vi "NMRvmeCard4.vi"() -> ()   [LabVIEW 2013]
uses:
  <vilib>/Utility/file.llb/Read From Spreadsheet File (DBL).vi
  <vilib>/Analysis/NI_AALBase.lvlib
panel:
  out "Peak center (MHz)":sgl=213.00728 format="%.3f"
  out "Peak width (MHz)":sgl=0.03243152 format="%.5f"
  in  "Max":bool=TRUE
  in  "Logoffset (V)":dbl=-5.924000000000002 min=-9.0 max=0.0 step=0.0005 format="%_5g"
  in  "Phase (V)":dbl=6.5 min=0.0 max=9.0 step=0.0005 format="%_5g"
  out "Telnet error out":errorcluster
  in  "Real/Quad Q curve":bool
  out "Temperature (C)":dbl(graph)=25.12
  out "+3V supply":dbl=3.245 format="%_4g"
  out "Temp (C)":dbl=25.12 format="%_4g"
  in  "RemovePed":bool=TRUE
  in  "IF / LOG Det":bool
  in  "Q curve file":string="realback212a.txt"
  out "File name 2":string="C:\\users\\plm\\Desktop\\rssmt\\realback212a.txt"
  in  "AutoTune":bool
  out "RF OK":bool=TRUE
  out "Peak area (V-MHz)":sgl=0.030005611 format="%.5f"
  in  "Gauss Fit":bool
  out "NMR Graph + Fit":cluster{cluster{dbl, "Numeric":dbl}[]}[](graph)=[{[{212.6, "Numeric"=-0.02921344062499997}, {212.60999999999999, "Numeric"=-0.03215714062499996}, {212.62, "Numeric"=-0.04651344062500006}, {212.63, "Numeric"=-0.03536254062499999}, {212.64, "Numeric"=-0.04138284062500002}, {212.65, "Numeric"=-0.041101840625000045}, {212.66, "Numeric"=-0.040491840625000046}, {212.67, "Numeric"=-0.026806840624999988}, {212.68, "Numeric"=-0.027852040624999956}, {212.69, "Numeric"=-0.040467640625000016}, {212.7, "Numeric"=-0.03304384062499998}, {212.71, "Numeric"=-0.031359340625}, {212.72, "Numeric"=-0.022591940624999994}, {212.73, "Numeric"=-0.01193064062500001}, {212.74, "Numeric"=-0.01354794062499997}, {212.75, "Numeric"=-0.013213040624999998}, {212.76, "Numeric"=-0.015344740624999985}, {212.77, "Numeric"=-0.00963054062500001}, {212.78, "Numeric"=-0.01998944062499996}, {212.79, "Numeric"=-0.029504540624999985}, {212.8, "Numeric"=-0.024544640624999982}, {212.81, "Numeric"=-0.024524280624999985}, {212.82, "Numeric"=-0.03563309062499998}, {212.82999999999998, "Numeric"=-0.027916150624999976}, {212.84, "Numeric"=-0.024776840624999984}, {212.85, "Numeric"=-0.018898880624999982}, {212.85999999999999, "Numeric"=-0.029138710624999974}, {212.87, "Numeric"=-0.028821390624999978}, {212.88, "Numeric"=-0.020467430624999977}, {212.89, "Numeric"=-0.017315150624999977}, {212.9, "Numeric"=-0.01772434062499998}, {212.91, "Numeric"=-0.01372252062499998}, {212.92, "Numeric"=-0.004970290624999978}, {212.93, "Numeric"=0.006207539375000022}, {212.94, "Numeric"=0.027450659375000026}, {212.95, "Numeric"=0.06105685437500003}, {212.96, "Numeric"=0.124804897375}, {212.97, "Numeric"=0.208860369375}, {212.98, "Numeric"=0.347462365375}, {212.99, "Numeric"=0.35238067957499997}, {213.0, "Numeric"=0.27427406967500007}, {213.01, "Numeric"=0.235365305375}, {213.02, "Numeric"=0.19710875937500003}, {213.03, "Numeric"=0.155801636375}, {213.04, "Numeric"=0.14391716037500002}, {213.05, "Numeric"=0.15687335037500003}, {213.06, "Numeric"=0.14626102237500002}, {213.07, "Numeric"=0.16260765937500002}, {213.08, "Numeric"=0.140506499375}, {213.09, "Numeric"=0.098470809375}, {213.1, "Numeric"=0.06081699937500002}, {213.11, "Numeric"=0.04152627937500002}, {213.12, "Numeric"=0.044080989375000025}, {213.13, "Numeric"=0.02363172937500002}, {213.14000000000001, "Numeric"=0.030902539375000024}, {213.15, "Numeric"=0.04097138937500002}, {213.16, "Numeric"=0.04776892937500001}, {213.17000000000002, "Numeric"=0.059566619375000025}, {213.18, "Numeric"=0.058962209375}, {213.19, "Numeric"=0.03914579937500002}, {213.2, "Numeric"=0.03482955937500002}, {213.21, "Numeric"=0.037365659375000006}, {213.22, "Numeric"=0.016002559375000038}, {213.23, "Numeric"=0.013610259374999996}, {213.24, "Numeric"=0.023504359375000013}, {213.25, "Numeric"=0.020751659374999988}, {213.26, "Numeric"=0.014210559374999994}, {213.27, "Numeric"=0.01739725937500001}, {213.28, "Numeric"=0.023614959374999973}, {213.29, "Numeric"=0.018911459375000002}, {213.3, "Numeric"=0.023336959374999973}, {213.31, "Numeric"=0.02134245937500002}, {213.32, "Numeric"=0.017474059375000024}, {213.33, "Numeric"=0.018297259374999993}, {213.34, "Numeric"=0.013561559374999983}, {213.35, "Numeric"=0.02328705937499998}, {213.36, "Numeric"=0.021839359374999985}, {213.37, "Numeric"=0.031837559375}, {213.38, "Numeric"=0.038417959374999984}, {213.39000000000001, "Numeric"=0.04150235937499997}, {213.4, "Numeric"=0.04535425937499999}]}]
  in  "Amp of Q curve":dbl=1.1 min=0.0 max=9.0 step=0.01 format="%_3f"
  in  "Subtract Q curve":bool=TRUE
  out "Pedestal Offset":dbl(graph)=0.028833440624999977
  out "Pedestal Difference":dbl(graph)=0.056176981249999994
  out "# Good Spectra":i32=994
  in  "Quality cuts":bool=TRUE
  out "Pedestal OK":bool=TRUE
  out "Sweep #":i32=6
  out "1st Sweep":bool
  out "ADC volts OK":bool=TRUE
  out "Peak Height Distribution":cluster{"Y":dbl[], "Y":dbl[]}[](graph)=[{"Y"=[0.6224574999999992, 0.6237974999999992, 0.6251374999999992, 0.6264774999999992, 0.6278174999999993, 0.6291574999999993, 0.6304974999999993, 0.6318374999999993, 0.6331774999999993, 0.6345174999999993, 0.6358574999999993, 0.6371974999999993, 0.6385374999999993, 0.6398774999999993, 0.6412174999999992, 0.6425574999999992, 0.6438974999999992, 0.6452374999999992, 0.6465774999999993, 0.6479174999999993, 0.6492574999999993, 0.6505974999999993, 0.6519374999999993, 0.6532774999999993, 0.6546174999999993, 0.6559574999999993, 0.6572974999999993, 0.6586374999999993, 0.6599774999999993, 0.6613174999999992, 0.6626574999999992, 0.6639974999999992, 0.6653374999999992, 0.6666774999999993, 0.6680174999999993, 0.6693574999999993, 0.6706974999999993, 0.6720374999999993, 0.6733774999999993, 0.6747174999999993, 0.6760574999999993, 0.6773974999999993, 0.6787374999999993, 0.6800774999999992, 0.6814174999999992, 0.6827574999999992, 0.6840974999999992, 0.6854374999999993, 0.6867774999999993, 0.6881174999999993, 0.6894574999999993, 0.6907974999999993, 0.6921374999999993, 0.6934774999999993, 0.6948174999999993, 0.6961574999999993, 0.6974974999999993, 0.6988374999999992, 0.7001774999999992, 0.7015174999999992, 0.7028574999999992, 0.7041974999999993, 0.7055374999999993, 0.7068774999999993, 0.7082174999999993, 0.7095574999999993, 0.7108974999999993, 0.7122374999999993, 0.7135774999999993, 0.7149174999999993, 0.7162574999999993, 0.7175974999999993, 0.7189374999999992, 0.7202774999999992, 0.7216174999999992, 0.7229574999999993, 0.7242974999999993, 0.7256374999999993, 0.7269774999999993, 0.7283174999999993, 0.7296574999999993, 0.7309974999999993, 0.7323374999999993, 0.7336774999999993, 0.7350174999999993, 0.7363574999999993, 0.7376974999999992, 0.7390374999999992, 0.7403774999999992, 0.7417174999999993, 0.7430574999999993, 0.7443974999999993, 0.7457374999999993, 0.7470774999999993, 0.7484174999999993, 0.7497574999999993, 0.7510974999999993, 0.7524374999999993, 0.7537774999999993, 0.7551174999999993], "Y"=[1.0, 0.0, 1.0, 0.0, 5.0, 2.0, 5.0, 1.0, 3.0, 2.0, 5.0, 1.0, 2.0, 1.0, 6.0, 4.0, 5.0, 4.0, 7.0, 3.0, 5.0, 6.0, 10.0, 7.0, 9.0, 12.0, 14.0, 12.0, 11.0, 17.0, 15.0, 8.0, 16.0, 15.0, 19.0, 16.0, 18.0, 16.0, 17.0, 12.0, 14.0, 16.0, 12.0, 17.0, 17.0, 22.0, 24.0, 20.0, 21.0, 21.0, 13.0, 20.0, 24.0, 17.0, 15.0, 13.0, 19.0, 20.0, 21.0, 20.0, 15.0, 18.0, 16.0, 15.0, 18.0, 15.0, 16.0, 18.0, 14.0, 15.0, 8.0, 9.0, 11.0, 4.0, 10.0, 6.0, 10.0, 10.0, 7.0, 11.0, 6.0, 6.0, 6.0, 4.0, 5.0, 5.0, 4.0, 7.0, 3.0, 3.0, 7.0, 3.0, 1.0, 1.0, 3.0, 1.0, 0.0, 1.0, 2.0, 1.0]}]
  in  "# of Sweeps":i32=1000
  out "S/N":dbl=26.28655612411849 format="%_3g"
  out "Peak mean (V)":dbl=0.6892010010060354 format="%_4g"
  out "Peak Height":dbl(graph)=0.35238067957499997
  in  "Raw Data":bool=TRUE
  in  "Tank RF":bool=TRUE
  in  "IF Atten (dB)":i8=4 min=0 max=31 step=1
  in  "IFoffset (V)":dbl=6.585236000000003 min=-0.0 max=9.0 step=0.001 format="%.4f"
  in  "Tune  (V)":dbl=1.1010000000000049 min=-0.5 max=8.0 step=0.001 format="%.4f"
  in  "Hi / Lo Gain":bool
  out "Voltage Array":sgl[](array[numeric])=[0.4262, 0.4197, 0.3847, 0.3757, 0.3504, 0.3312, 0.313, 0.3087, 0.2902, 0.2602, 0.2515, 0.2368, 0.2298, 0.2253, 0.2091, 0.1954, 0.1799, 0.1725, 0.1496, 0.1277, 0.1211, 0.1102, 0.0891, 0.0869, 0.0805, 0.0772, 0.0592, 0.0512, 0.0524, 0.0492, 0.0427, 0.0407, 0.0448, 0.0521, 0.0689, 0.099, 0.1599, 0.2418, 0.3788, 0.3818, 0.3037, 0.2653, 0.2277, 0.1881, 0.1781, 0.193, 0.1854, 0.2053, 0.187, 0.15, 0.1177, 0.1043, 0.1138, 0.1002, 0.1148, 0.1335, 0.1487, 0.1693, 0.1785, 0.1695, 0.1766, 0.1914, 0.1826, 0.1934, 0.2169, 0.2284, 0.2366, 0.2553, 0.2779, 0.2899, 0.3117, 0.3284, 0.3435, 0.364, 0.3796, 0.41, 0.4299, 0.4615, 0.491, 0.5174, 0.5452] format="%.4f"
  in  "Invert Polarity":bool=TRUE
  out "Pedestal Diff (V)":sgl=0.056176983 format="%.3f"
  out "Peak amp (V)":sgl=0.3523807 format="%.3f"
  in  "Save Data to File":bool
  in  "RF Level (dBm)":dbl min=-10.0 max=10.0 step=0.1 format="%.2f"
  out "SMT error out":errorcluster
  out "Sample RMS (V)":dbl=0.009830864197530865 format="%.4f"
  in  "# Sample/step":i32=80 min=1 max=5000 step=100
  in  "Step Width (MHz)":dbl=0.01 min=0.0 max=1000.0 step=0.0005 format="%.4f"
  in  "Freq Span (MHz)":dbl=0.8 min=0.0 max=3000.0 step=0.1 format="%.3f"
  in  "Center Freq (MHz)":dbl=213.0 min=0.005 max=6000.0 step=0.1 format="%.3f"
  in  "Sweep Mode":u16(ring)=3 items=["Off", "Single", "Auto", "Step"]
  in  "GPIB Addr (28)":refnum<visa-resource-name>="GPIB0::28::INSTR"
  # "E1039 Prototype NMR Control Panel"
  # "Settings"
  # "D\nA\nC"
  # "R\nF\n\nG\nE\nN \n\n+\n\nI\nF"
  # "A\nD\nC"
  # "I\n/\nO"
  # "D\nA\nT\nA\n\nA \nN\nA\nL\nY\nS\nI\nS"
  # "Results"
  # "A\nv\ne\nr\na\ng\ne"
  # "S\nw\ne\ne\np"
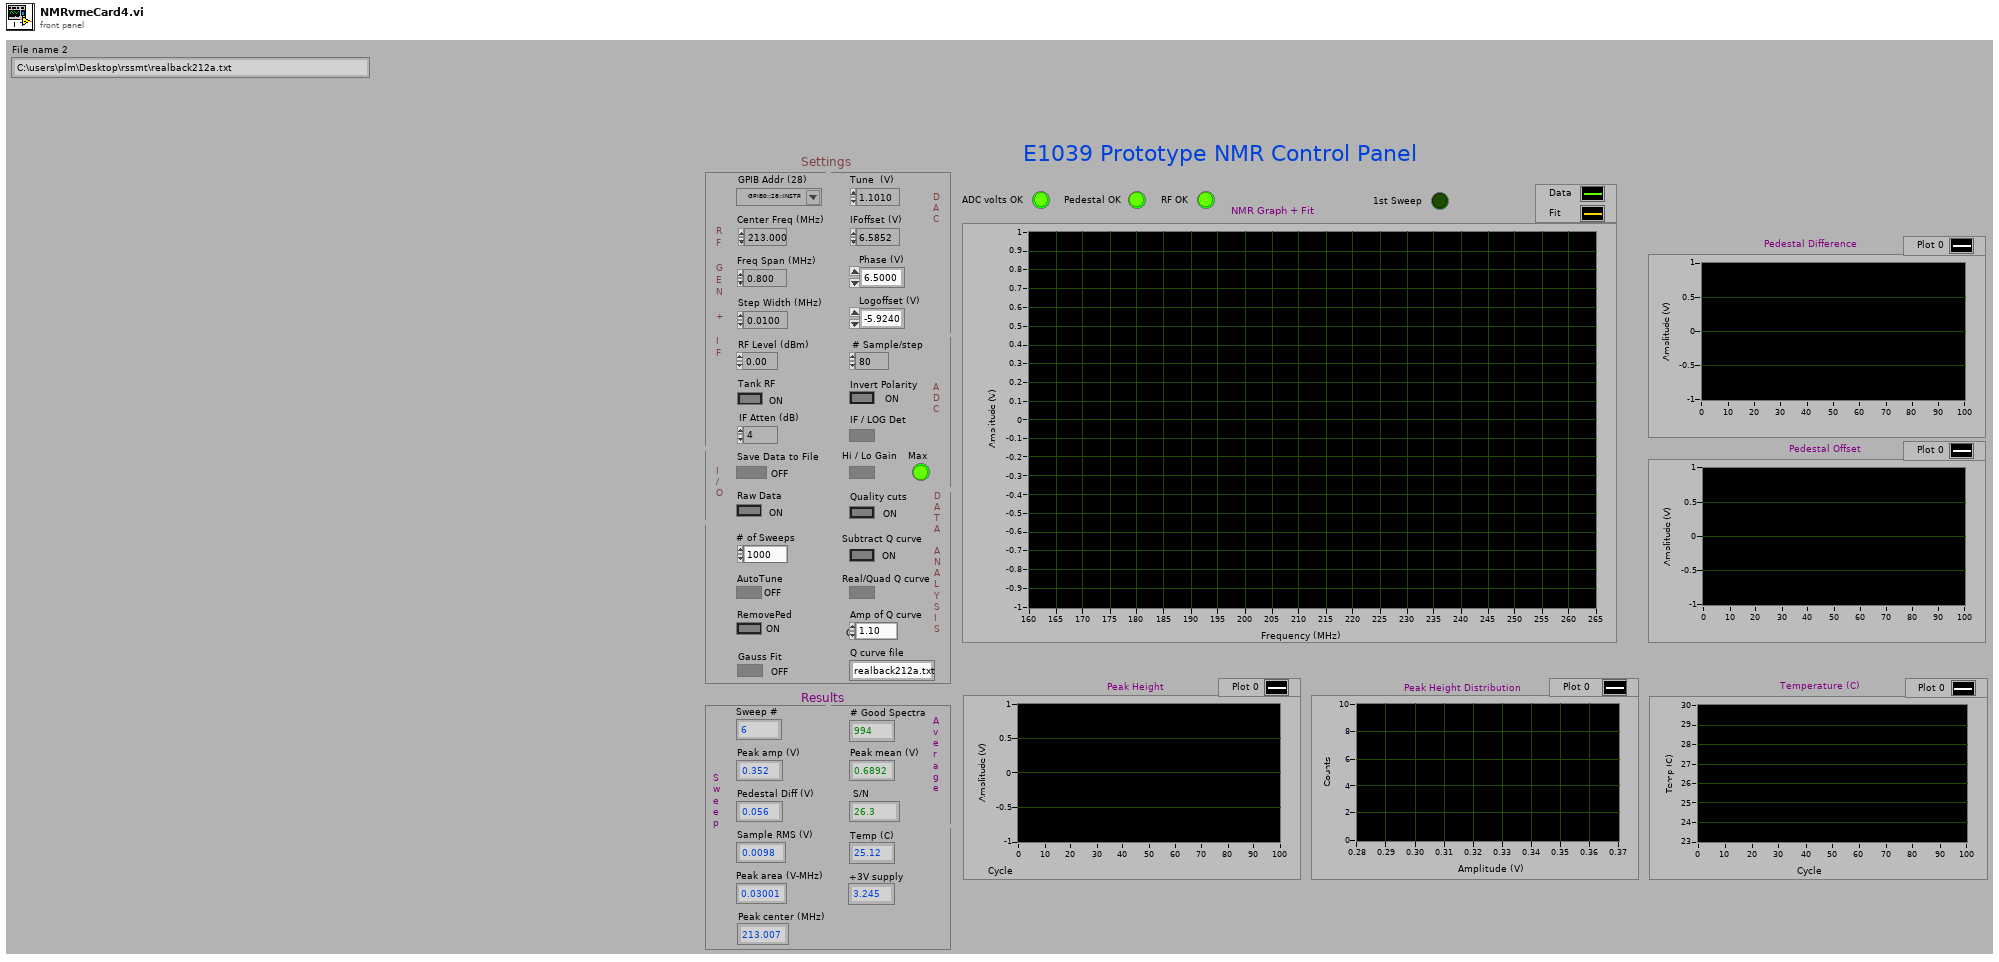
[diagram p1: front panel]
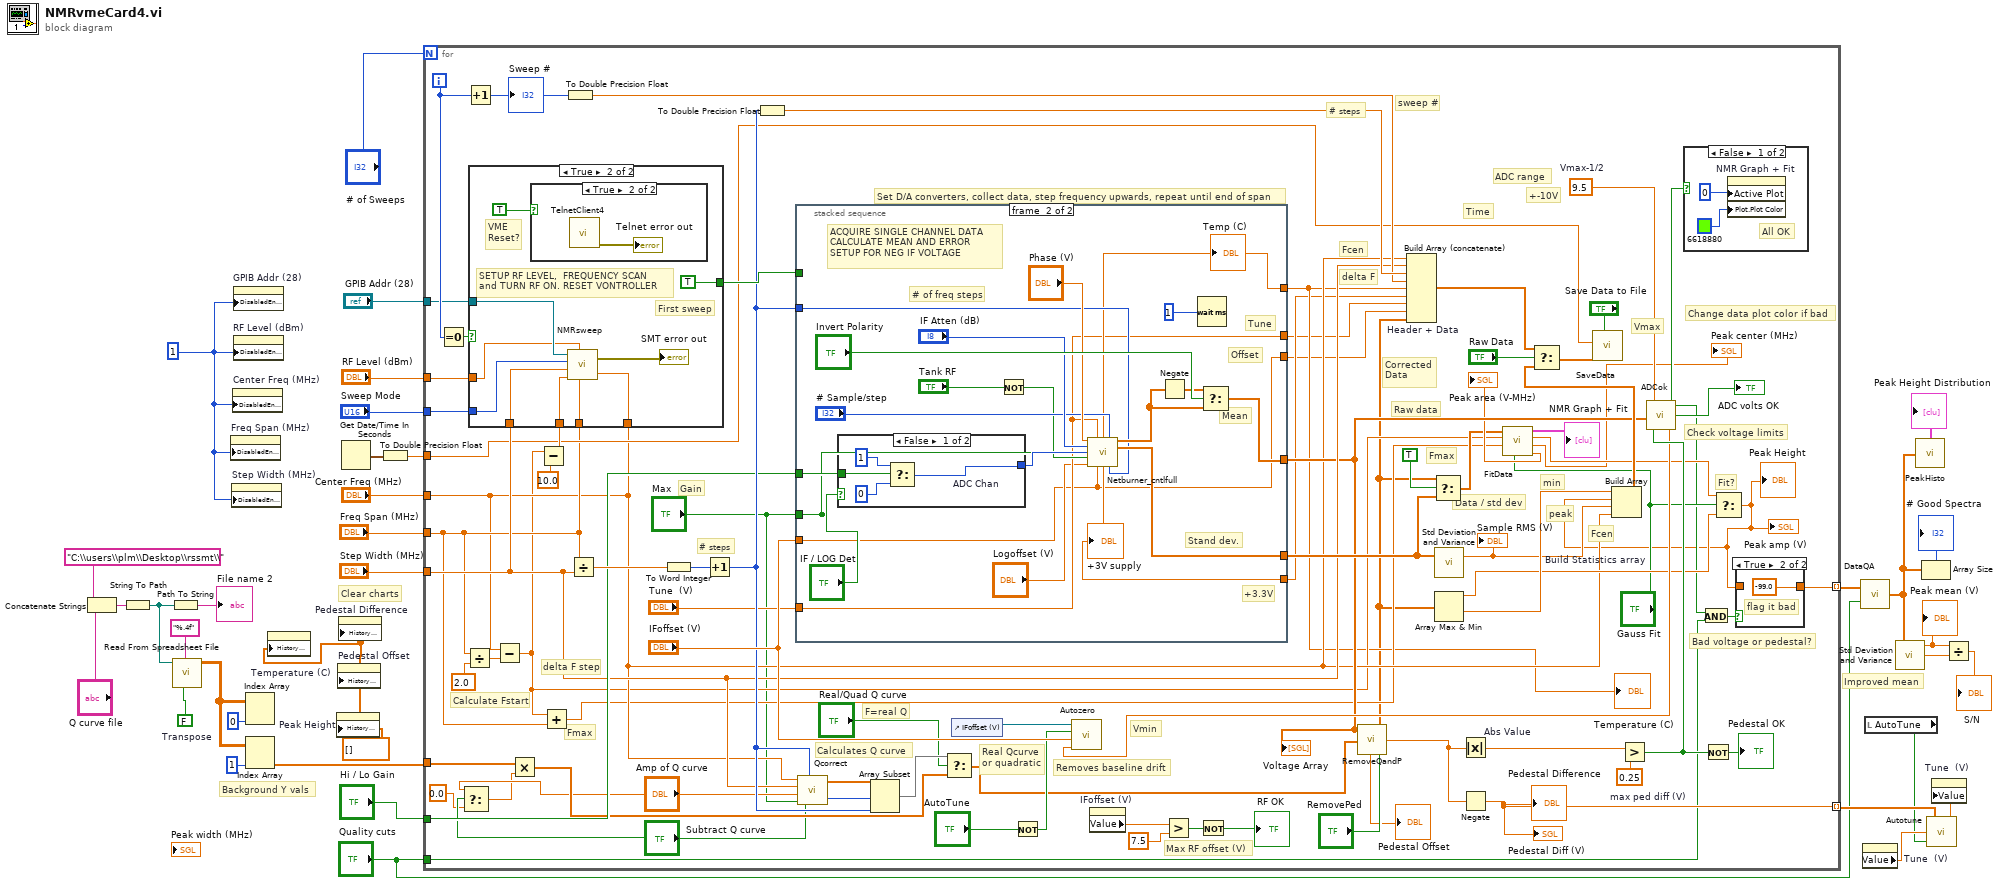
[diagram p0: block diagram]
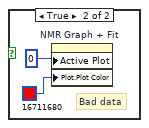
[diagram p2: hidden frame]
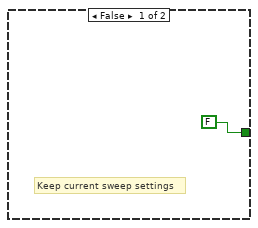
[diagram p4: hidden frame]
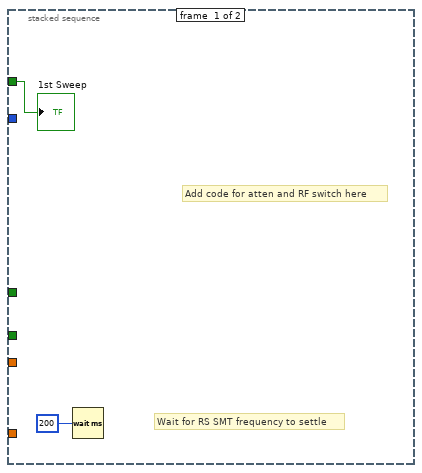
[diagram p6: hidden frame]
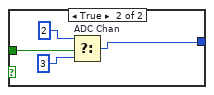
[diagram p7: hidden frame]
diagram:
  w2 = 1
  w14 = FALSE  # Transpose
  w6 = dbl[] []
  # "Background Y vals"
  # "Clear charts"
  # "Improved mean"
  n1 = Concatenate Strings "Concatenate Strings"("C:\\users\\plm\\Desktop\\rssmt\\", "Q curve file") -> (w17:string)
  n2 = String To Path(string=w17) -> (path=w13:path)
  n3 = Path To String(path=w13) -> (string=→"File name 2":string)
  n4 = call-poly <vilib>:"Read From Spreadsheet File.vi"("transpose (no:F)"=w14, "format (%.3f)"="%.4f", "file path (dialog if empty)"=w13) -> ("all rows"=w12:dbl[][])  [unwired: 4 in, 4 out]
  n5 = property on="Freq Span (MHz)" class="DigNum (strict)"("DisabledEnum"=w2) -> ()  [unwired: 2 in, 2 out]
  n6 = property on="Step Width (MHz)" class="DigNum (strict)"("DisabledEnum"=w2) -> ()  [unwired: 2 in, 2 out]
  n7 = property on="Center Freq (MHz)" class="DigNum (strict)"("DisabledEnum"=w2) -> ()  [unwired: 2 in, 2 out]
  n8 = property on="GPIB Addr (28)" class="VISAName"("DisabledEnum"=w2) -> ()  [unwired: 2 in, 2 out]
  n9 = property on="RF Level (dBm)" class="DigNum (strict)"("DisabledEnum"=w2) -> ()  [unwired: 2 in, 2 out]
  n10 = Index Array "Index Array"(array=w12, index (col)=0) -> ()  [unwired: 1 in, 1 out]
  n11 = Index Array(array=w12, index (col)=1) -> (element=w7:dbl[])  [unwired: 1 in]
  n12 = property on="Temperature (C)" class="WFChart (strict)"("History Data"=w6) -> ()  [unwired: 2 in, 2 out]
  n13 = property on="Peak Height" class="WFChart (strict)"("History Data"=w6) -> ()  [unwired: 2 in, 2 out]
  n14 = property on="Pedestal Offset" class="WFChart (strict)"("History Data"=w6) -> ()  [unwired: 2 in, 2 out]
  n15 = property on="Pedestal Difference" class="WFChart (strict)"("History Data"=w6) -> ()  [unwired: 2 in, 2 out]
  n16 = Get Date/Time In Seconds() -> (seconds since 1Jan1904=w19:timestamp)
  n17 = To Double Precision Float(number=w19) -> (double precision float=w18:dbl)
  n18 = for {
    N: "# of Sweeps" -> [_]
    tunnel: [w101] -> w33 mode=indexing
    tunnel: "Quality cuts" -> [w79]
    tunnel: [w85] -> w30 mode=indexing
    tunnel: "Center Freq (MHz)" -> [w66]
    tunnel: "Freq Span (MHz)" -> [w72]
    tunnel: "Step Width (MHz)" -> [w78]
    tunnel: "Sweep Mode" -> [w89]
    tunnel: "Hi / Lo Gain" -> [w88]
    tunnel: "GPIB Addr (28)" -> [w87]
    tunnel: "RF Level (dBm)" -> [w86]
    tunnel: w18 -> [w73]
    tunnel: w7 -> [w51]
    i -> [w99]
    w83 = 9.5  # Vmax-1/2
    w102 = 0.25  # max ped diff (V)
    # "Gain"
    # "F=real Q"
    # "Real Qcurve\nor quadratic"
    # "+-10V"
    # "Vmax"
    # "Change data plot color if bad"
    # "Max RF offset (V)"
    # "Fmax"
    # "Fit?"
    # "Fmax"
    # "Time"
    # "Vmin"
    # "min"
    # "peak"
    # "Raw data"
    # "Corrected\nData"
    # "Fcen"
    # "delta F"
    # "# steps"
    # "ADC range"
    # "sweep #"
    # "Fcen"
    # "Set D/A converters, collect data, step frequency upwards, repeat until end of span"
    # "Calculates Q curve"
    # "Removes baseline drift"
    # "Bad voltage or pedestal?"
    # "Check voltage limits"
    # "Data / std dev"
    # "# steps"
    # "Calculate Fstart"
    # "delta F step"
    n19 = Equal To 0?(x=w99) -> (x = 0?=w104:bool)
    n20 = Select(t="Amp of Q curve", s="Subtract Q curve", f=0.0) -> (s? t:f=w46:dbl)
    n21 = Divide(x=w72, y=sgl 2.0) -> (x/y=w115:dbl)
    n22 = Increment(x=w99) -> (x+1=w90:i32)
    "Sweep #" <- w90
    n23 = Subtract(x=w66, y=w115) -> (x-y=w61:dbl)
    n24 = Multiply(x=w51, y=w46) -> (x*y=w50:dbl[])
    n25 = Subtract(x=w61, y=10.0) -> (x-y=w113:dbl)
    n26 = case shown="True" w104 {
      tunnel: w113 -> [_ w134]
      tunnel: w78 -> [_ w132]
      tunnel: w66 -> [_ w131]
      tunnel: w72 -> [_ w133]
      tunnel: [FALSE TRUE] -> w103
      tunnel: w89 -> [_ w128]
      tunnel: w87 -> [_ w127]
      tunnel: w86 -> [_ w126]
      frame False {
        # "Keep current sweep settings"
      }
      frame True {
        # "VME\nReset?"
        # "First sweep"
        # "SETUP RF LEVEL,  FREQUENCY SCAN\nand TURN RF ON. RESET VONTROLLER"
        n27 = case shown="True" TRUE {
          frame False {
          }
          frame True {
            n28 = call "TelnetClient4.vi"() -> ("Telnet error"=→"Telnet error out":errorcluster)  [unwired: 4 in, 3 out]
          }
        }
        n29 = call "NMRsweep.vi"("Center Freq (MHz)"=w131, "Freq Span (MHz)"=w133, "RF Level (dBm)"=w126, "Foffset (MHz)"=w134, "Step Width (MHz)"=w132, "Sweep Mode"=w128, "GPIB Addr (28)"=w127) -> ("error out"=→"SMT error out":errorcluster)
      }
    }
    n30 = Add(x=w61, y=w72) -> (x+y=w60:dbl)
    n31 = To Double Precision Float(number=w90) -> (double precision float=w91:dbl)
    n32 = Divide(x=w72, y=w78) -> (x/y=w117:dbl)
    n33 = To Word Integer(number=w117) -> (16bit integer=w114:i16)
    n34 = Increment(x=w114) -> (x+1=w93:i16)
    n35 = To Double Precision Float(number=w93) -> (double precision float=w92:dbl)
    n36 = stacked-sequence {
      tunnel: [_ w149] -> w107
      tunnel: [_ w156] -> w76
      tunnel: w93 -> [_ w146]
      tunnel: "IFoffset (V)" -> [_ w139]
      tunnel: w88 -> [_ w154]
      tunnel: w103 -> [w136 _]
      tunnel: "Tune  (V)" -> [_ w141]
      tunnel: [_ w145] -> w42
      tunnel: [_ w142] -> w41
      tunnel: [_ w141] -> w39
      tunnel: [_ w139] -> w38
      tunnel: [_ w138] -> _
      tunnel: "Max" -> [_ w138]
      frame #0 {
        # "Add code for atten and RF switch here"
        # "Wait for RS SMT frequency to settle"
        n37 = Wait (ms)(milliseconds to wait=200) -> ()  [unwired: 1 out]
        "1st Sweep" <- w136
      }
      frame #1 {
        # "+3.3V"
        # "Offset"
        # "Tune"
        # "Stand dev."
        # "Mean"
        # "ACQUIRE SINGLE CHANNEL DATA\nCALCULATE MEAN AND ERROR\nSETUP FOR NEG IF VOLTAGE"
        # "# of freq steps"
        n38 = case shown="False" "IF / LOG Det" {
          tunnel: w154 -> [w162 w163]
          tunnel: [w159 w164] -> w148
          frame False {
            n39 = Select "ADC Chan"(t=1, s=w162, f=0) -> (s? t:f=w159:i32)
          }
          frame True {
            n40 = Select "ADC Chan"(t=2, s=w163, f=3) -> (s? t:f=w164:i32)
          }
        }
        n41 = Not(x="Tank RF") -> (.not. x?=w144:bool)
        n42 = call "Netburner_cntlfull.vi"("Phase Volt"="Phase (V)", "Tune Volt"=w141, "# Data"="# Sample/step", "IF Atten (dB)"="IF Atten (dB)", "NMR ADC"=w148, "Hi Gain"=w138, "Tank RF"=w144, "LogOff Volt"="Logoffset (V)", "IFOff Volt"=w139, "# f steps"=w146) -> ("Temp (C)"=w145:dbl, "ADC value"=w150:dbl[], "ADC error"=w149:dbl[], "Volts"=w142:dbl)  [unwired: 2 out]
        "Temp (C)" <- w145
        "+3V supply" <- w142
        n43 = Negate(x=w150) -> (-x=w155:dbl[])
        n44 = Wait (ms)(milliseconds to wait=1) -> ()  [unwired: 1 out]
        n45 = Select(t=w155, s="Invert Polarity", f=w150) -> (s? t:f=w156:dbl[])
      }
    }
    "Voltage Array" <- w76
    "Temperature (C)" <- w42
    n46 = call "Qcorrect.vi"("Subtract Q curve"="Subtract Q curve", "Nstep"=w93, "Max Gain"="Max", "Amp of Q curve"="Amp of Q curve", "Step Width (MHz)"=w78, "Center Freq (MHz)"=w66) -> ("Start"=w108:i32, "Array"=w109:dbl[])
    n47 = Array Subset "Array Subset"(array=w109, index=w108, length=w93) -> (w54:dbl[])
    n48 = Select(t=w54, s="Real/Quad Q curve", f=w50) -> (s? t:f=w53:dbl[])
    n49 = control-ref of="IFoffset (V)"() -> (w82:refnum<vi>)
    n50 = Not(x="AutoTune") -> (.not. x?=w55:bool)
    n51 = property on="IFoffset (V)" class="DigNum (strict)"() -> ("Value"=w70:dbl)  [unwired: 2 in, 2 out]
    n52 = Greater?(x=w70, y=7.5) -> (0:w68:bool)
    n53 = Not(x=w68) -> (.not. x?=→"RF OK":bool)
    n54 = call "RemoveQandP.vi"("Subtract Ped?"="RemovePed", "Qcurve"=w53, "Raw data"=w76) -> ("Ped L-R"=w95:dbl, "Corrected data"=w40:dbl[], "Ped Offfset"=→"Pedestal Offset":dbl)
    n55 = Build Array (concatenate) "Header + Data"(w66, w78, w92, w91, w42, w41, w39, w38, w40) -> (w94:dbl[])
    n56 = Select(t=w40, s=TRUE, f=w107) -> (s? t:f=w62:dbl[])
    n57 = call <vilib>:"Std Deviation and Variance.vi"("X"=w107) -> ("mean"=w77:dbl)  [unwired: 1 in, 2 out]
    "Sample RMS (V)" <- w77
    n58 = Array Max & Min(array=w40) -> (max value=w71:dbl, min value=w106:dbl)  [unwired: 2 out]
    n59 = Absolute Value "Abs Value"(x=w95) -> (abs(x)=w97:dbl)
    n60 = Negate(x=w95) -> (-x=w85:dbl)
    "Pedestal Diff (V)" <- w85
    "Pedestal Difference" <- w85
    n61 = call "FitData.vi"("Fit?"="Gauss Fit", "Fmax"=w60, "Fmin"=w61, "Yarray"=w62) -> ("Peak Area (V-MHz)"=→"Peak area (V-MHz)":dbl, "Center Freq (MHz)"=→"Peak center (MHz)":dbl, "Amplitude (V)"=w64:dbl, "NMR Graph + Fit"=→"NMR Graph + Fit":cluster{cluster{dbl, "Numeric":dbl}[]}[])  [unwired: 1 out]
    n62 = Greater?(x=w97, y=w102) -> (0:w84:bool)
    n63 = call "ADCok.vi"("PedOK"=w84, "Array"=w76, "Vmax-1/2"=w83) -> ("Vmin"=w81:dbl, "ADC voltages OK"=→"ADC volts OK":bool, "Allok"=w58:bool)
    n64 = call "Autozero.vi"("Vmin (V)"=w81, "IFoffset (V)"="IFoffset (V)", "Enable"=w55, "reference"=w82) -> ()
    n65 = case shown="False" w58 {
      frame False {
        # "All OK"
        n66 = property on="NMR Graph + Fit" class="XYGraph (strict)"("Active Plot"=0, "Plot.Plot Color"=u32 6618880) -> ()  [unwired: 2 in, 2 out]
      }
      frame True {
        # "Bad data"
        n67 = property on="NMR Graph + Fit" class="XYGraph (strict)"("Active Plot"=0, "Plot.Plot Color"=u32 16711680) -> ()  [unwired: 2 in, 2 out]
      }
    }
    n68 = And(x=w58, y=w79) -> (x .and. y?=w98:bool)
    n69 = Not(x=w84) -> (.not. x?=→"Pedestal OK":bool)
    n70 = Select(t=w64, s="Gauss Fit", f=w71) -> (s? t:f=w57:dbl)
    "Peak amp (V)" <- w57
    "Peak Height" <- w57
    n71 = Build Array "Build Statistics array"(w106, w57, w77, w66) -> (w112:dbl[])
    n72 = Select(t=w94, s="Raw Data", f=w112) -> (s? t:f=w74:dbl[])
    n73 = call "SaveData.vi"("Array"=w74, "Save Data to File"="Save Data to File", "Ext time (sec)"=w73) -> ()  [unwired: 1 out]
    n74 = case shown="True" w98 {
      tunnel: [w122 -99.0] -> w101
      tunnel: w57 -> [w122 _]
      frame False {
        # "Data OK"
      }
      frame True {
        # "flag it bad"
      }
    }
  }
  n75 = call "DataQA.vi"("Quality cuts"="Quality cuts", "Data In"=w33) -> ("Data Out"=w32:dbl[])
  n76 = property on="Tune  (V)" class="DigNum (strict)"() -> ("Value"=w22:dbl)  [unwired: 2 in, 2 out]
  n77 = local read "AutoTune"() -> (w1:bool)
  n78 = call <vilib>:"Std Deviation and Variance.vi"("X"=w32) -> ("mean"=w5:dbl, "standard deviation"=w4:dbl)  [unwired: 1 in, 1 out]
  "Peak mean (V)" <- w5
  n79 = call "PeakHisto.vi"("Data Out"=w32) -> ("XY Graph"=→"Peak Height Distribution":cluster{"Y":dbl[], "Y":dbl[]}[])
  n80 = Array Size(array=w32) -> (size(s)=→"# Good Spectra":i32)
  n81 = call "Autotune.vi"("Adjust Tune"=w1, "Tune Vin"=w22, "Pedestal Diff"=w30) -> ("Tune Vout"=w21:dbl)
  n82 = property on="Tune  (V)" class="DigNum (strict)"("Value"=w21) -> ()  [unwired: 2 in, 2 out]
  n83 = Divide(x=w5, y=w4) -> (x/y=→"S/N":dbl)
